vi "Periodic Tasks.vi"(8 "error in":errorcluster) -> ()   [LabVIEW 2017]
doc: "This VI runs in parallel to other robot code. It can contain as many user-defined periodic loops as you need. These can carry out PID or other sorts of timed response."
uses:
  <vilib>/Rock Robotics/SystemInterfaces/spilib/spi_bus.ctl
  <vilib>/Rock Robotics/WPI/Utilities/WPI_GetSetVariantRefNum.vi
  <vilib>/Rock Robotics/WPI/Gyro/WPI_GyroXRS450_SPI_Open.vi
  <vilib>/Rock Robotics/Network Tables/NT Write Number.vi
  <vilib>/Rock Robotics/Network Tables/NT Write Numeric Array.vi
  Drive/Implementation/gyroNumControl.vi
panel:
  in  "SPI Bus":T1
  in  "Sample Rate (Hz)":dbl=1000.0 min=50.0 max=20000.0 format="%#_13g"
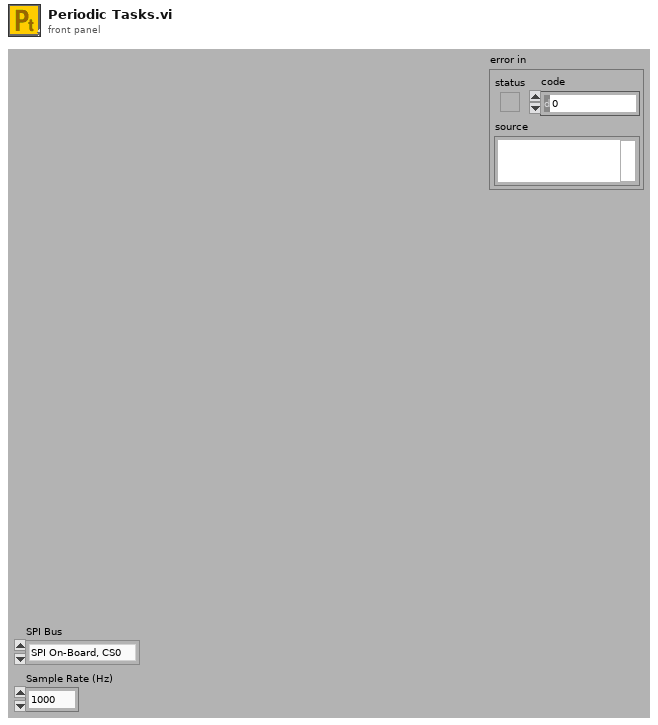
[diagram p1: front panel]
types:
  T1 = typedef "spi_bus.ctl" = enum16{"SPI On-Board, CS0", "SPI On-Board, CS1", "SPI On-Board, CS2", "SPI On-Board, CS3", "SPI MXP", "Invalid"}
  T2 = typedef "WPI_GyroDevRef.ctl" = cluster{"DevStatus":errorcluster, "Analog Channel":T3, "Gain (VoltsPerDegree/Second)":dbl, "Gyro Type":enum16{"Analog", "XRS450"}, "Handle":i32, "SPI Bus":T1, "Device Found":bool, "Sample Rate":dbl, "Calibrate On Open":bool, "Offset":dbl}
  T3 = typedef "FPGA_AIChannel.ctl" = enum8{"AI 0", "AI 1", "AI 2", "AI 3", "AI MXP 0", "AI MXP 1", "AI MXP 2", "AI MXP 3", "Invalid"}
  T4 = typedef "WPI_JoystickDevRef.ctl" = cluster{"Device":T5}
  T5 = typedef "WPI_JoystickDeviceEnum.ctl" = enum16{"USB 0", "USB 1", "USB 2", "USB 3", "USB 4", "USB 5"}
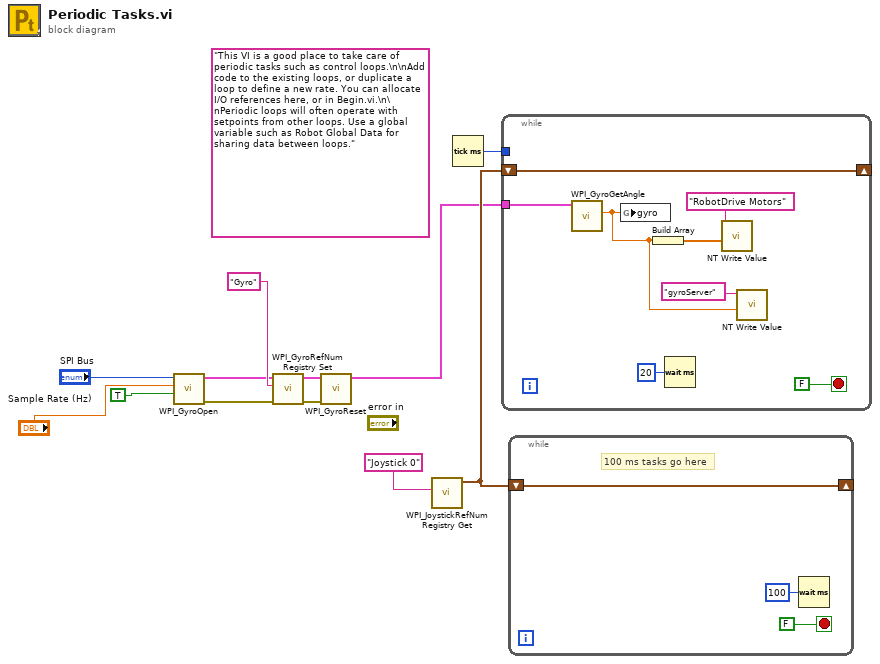
[diagram p0: block diagram]
diagram:
  (unwired) "This VI is a good place to take care of periodic tasks such as control loops.\n\nAdd code to the existing loops, or duplicate a loop to define a new rate. You can allocate I/O references here, or in Begin.vi.\n\nPeriodic loops will often operate with setpoints from other loops. Use a global variable such as Robot Global Data for sharing data between loops."
  n1 = call-poly <vilib>:"WPI_GyroOpen.vi"("Calibrate On Open"=TRUE, "Sample Rate (Hz)"="Sample Rate (Hz)", "SPI Bus"="SPI Bus") -> ("error out"=w5:errorcluster, "GyroDevRef"=w6:T2)  [unwired: 6 in, 1 out]
  n2 = call <vilib>:"WPI_GyroRefNum Registry Set.vi"("error in (no error)"=w5, "refnum name"="Gyro", "GyroDevRef"=w6) -> ("error out"=w2:errorcluster, "GyroDevRef"=w3:T2)  [unwired: 7 in]
  n3 = call <vilib>:"WPI_GyroReset.vi"("error in"=w2, "GyroDevRef"=w3) -> ("GyroDevRef"=w1:T2)  [unwired: 8 in, 1 out]
  n4 = call <vilib>:"WPI_JoystickRefNum Registry Get.vi"("refnum name"="Joystick 0") -> ("JoystickDevRef"=w11:T4)  [unwired: 1 in, 9 out]
  n5 = Tick Count (ms)() -> (millisecond timer value=w10:u32)
  n6 = while {
    shift-right: [w19] -> _
    shift-left: w11 -> [w19]
    tunnel: w10 -> [_]
    tunnel: w1 -> [w17]
    stop <- FALSE stop-if-true
    n7 = call <vilib>:"WPI_GyroGetAngle.vi"("GyroDevRef"=w17) -> ("Angle"=w14:dbl)  [unwired: 6 in, 4 out]
    n8 = global write "gyroNumControl.vi" "gyro"(w14) -> ()
    n9 = Build Array(w14) -> (w15:dbl[])
    n10 = Wait (ms)(milliseconds to wait=u32 20) -> ()  [unwired: 1 out]
    n11 = call-poly <vilib>:"NT Write Value.vi"("Numeric Array"=w15, "Name"="RobotDrive Motors") -> ()  [unwired: 9 in, 1 out]
    n12 = call-poly <vilib>:"NT Write Value.vi"("Numeric"=w14, "Name"="gyroServer") -> ()  [unwired: 9 in, 1 out]
  }
  n13 = while {
    shift-right: [w21] -> _
    shift-left: w11 -> [w21]
    stop <- FALSE stop-if-true
    # "100 ms tasks go here"
    n14 = Wait (ms)(milliseconds to wait=u32 100) -> ()  [unwired: 1 out]
  }
